vi "FRCts20_WebMethods_Convert_Request.vi"(8 "error in (no error)":errorcluster, 10 "Team Out":T8, 11 "Request Out":T9) -> (0 "error out":errorcluster, 3 "Request+Team":cluster{"Request":T1, "Team":T4})   [LabVIEW 2014, in "FRCts20_WebMethods.lvlib"]
uses:
  FRCts20_WebMethods.lvlib
  Backend/source/VI Source/FRCts20_Backend_API/FRCts20_Backend_API_Request.ctl
  Backend/source/VI Source/FRCts20_Backend_API/FRCts20_Backend_API_Status.ctl
  Backend/source/VI Source/FRCts20_Backend_API/FRCts20_Backend_API_Team.ctl
  Backend/source/VI Source/FRCts20_Backend_API/FRCts20_Backend_API_SW.ctl
  ESP Engine/source/VI Source/TypeDefs/FRCts20_EspEngine_Request.ctl
  Web Method Public Interface/FRCts20_WebMethods_ctl_request.ctl
  ESP Engine/source/VI Source/TypeDefs/FRCts20_EspEngine_Team.ctl
  Web Method Public Interface/FRCts20_WebMethods_ctl_singleTeam.ctl
  Web Method Public Interface/FRCts20_WebMethods_ctl_teamIdentifier.ctl
  ESP Engine/source/VI Source/FRCts20_EspEngine.lvlib
  Backend/source/VI Source/FRCts20_Backend_API/FRCts20_Backend_API.lvlib
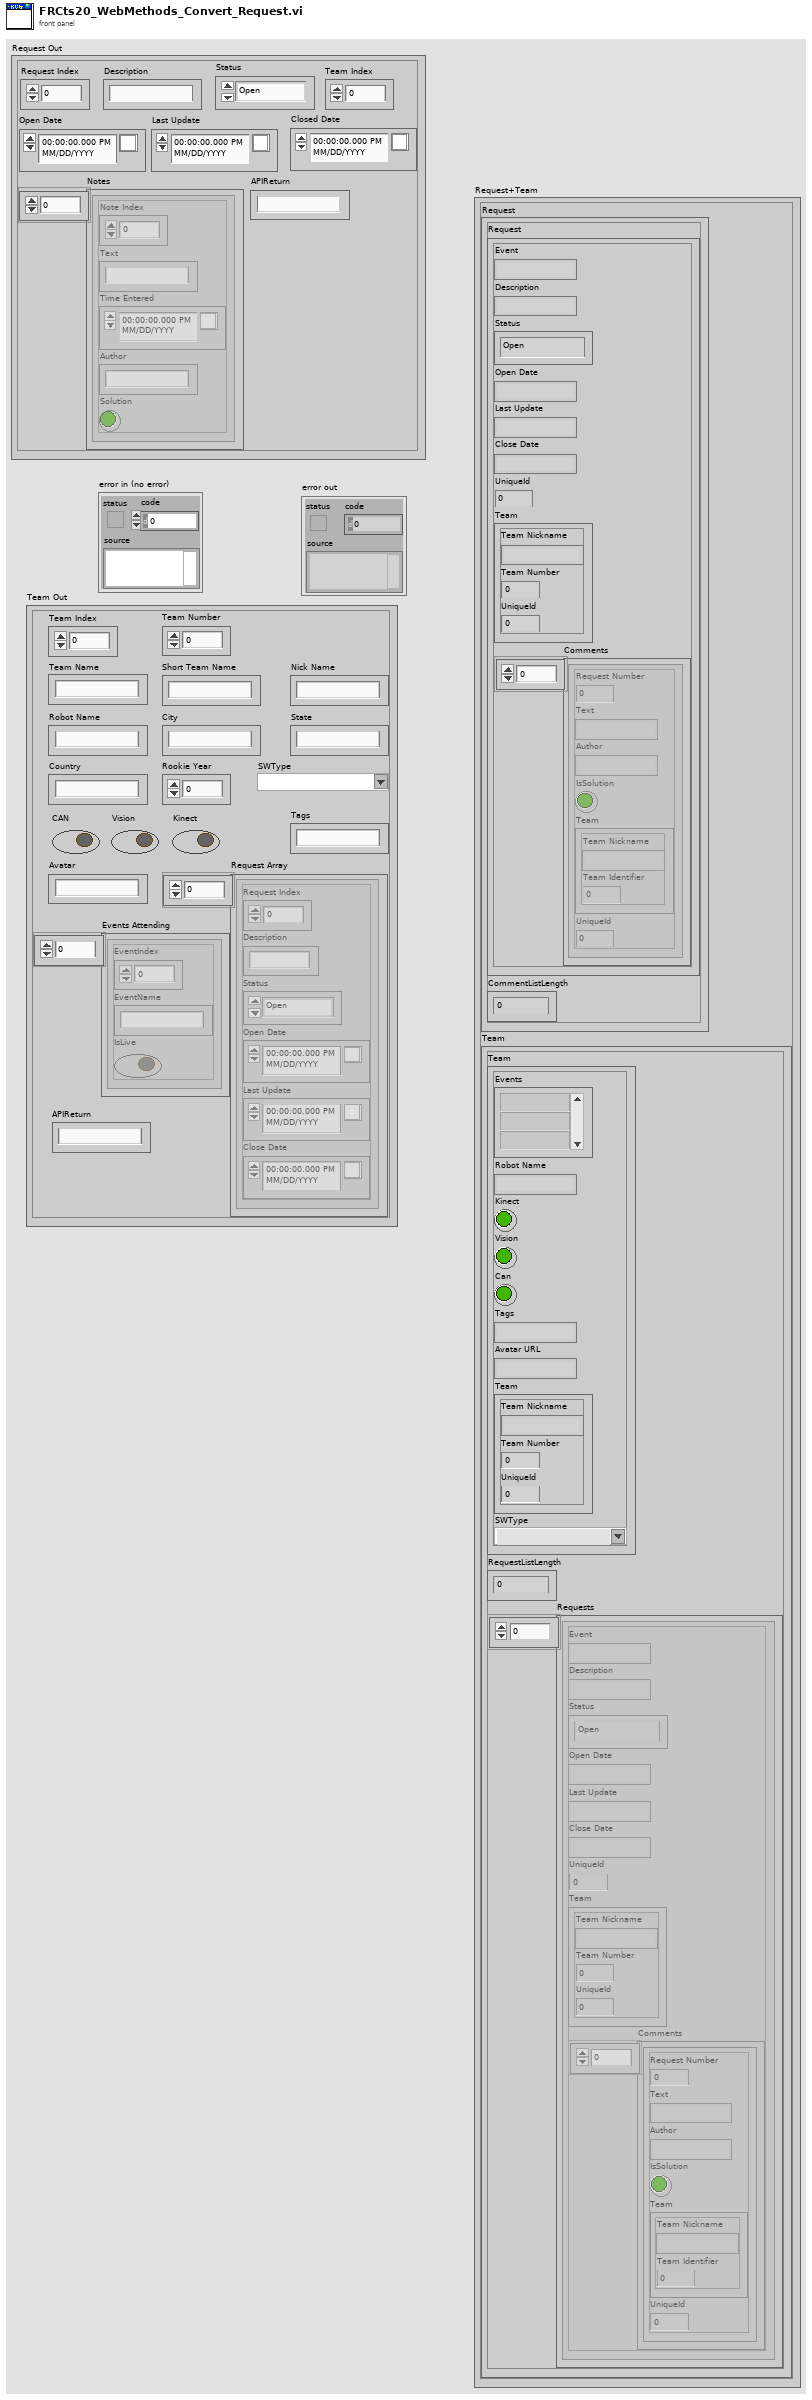
[diagram p1: front panel]
types:
  T1 = typedef "FRCts20_EspEngine.lvlib/FRCts20_EspEngine_Request.ctl" = cluster{"Request":T2, "CommentListLength":i16}
  T2 = typedef "FRCts20_WebMethods.lvlib/FRCts20_WebMethods_ctl_request.ctl" = cluster{"Event":string, "Description":string, "Status":T3, "Open Date":string, "Last Update":string, "Close Date":string, "UniqueId":i32, "Team":cluster{"Team Nickname":string, "Team Number ":i32, "UniqueId":i32}, "Comments":cluster{"Request Number":dbl, "Text":string, "Author":string, "IsSolution":bool, "Team":cluster{"Team Nickname":string, "Team Identifier ":dbl}, "UniqueId":i32}[]}
  T3 = typedef "FRCts20_Backend_Engine.lvlib/FRCts20_Backend_API.lvlib/FRCts20_Backend_API_Status.ctl" = enum16{"Open", "In Work", "Closed"}
  T4 = typedef "FRCts20_EspEngine.lvlib/FRCts20_EspEngine_Team.ctl" = cluster{"Team":T5, "RequestListLength":i16, "Requests":T2[]}
  T5 = typedef "FRCts20_WebMethods.lvlib/FRCts20_WebMethods_ctl_singleTeam.ctl" = cluster{"Events":string[], "Robot Name":string, "Kinect":bool, "Vision":bool, "Can":bool, "Tags":string, "Avatar URL":string, "Team":T6, "SWType":T7}
  T6 = typedef "FRCts20_WebMethods.lvlib/FRCts20_WebMethods_ctl_teamIdentifier.ctl" = cluster{"Team Nickname":string, "Team Number ":u32, "UniqueId":u32}
  T7 = typedef "FRCts20_Backend_Engine.lvlib/FRCts20_Backend_API.lvlib/FRCts20_Backend_API_SW.ctl" = string
  T8 = typedef "FRCts20_Backend_Engine.lvlib/FRCts20_Backend_API.lvlib/FRCts20_Backend_API_Team.ctl" = cluster{"Team Index":u32, "Team Number":u32, "Team Name":string, "Short Team Name":string, "Nick Name":string, "Robot Name":string, "City":string, "State":string, "Country":string, "Rookie Year":u32, "SWType":T7, "CAN":bool, "Vision":bool, "Kinect":bool, "Tags":string, "Avatar":string, "Request Array":cluster{"Request Index":u32, "Description":string, "Status":T3, "Open Date":timestamp, "Last Update":timestamp, "Close Date":timestamp}[], "Events Attending":cluster{"EventIndex":dbl, "EventName":string, "IsLive":bool}[], "APIReturn":string}
  T9 = typedef "FRCts20_Backend_Engine.lvlib/FRCts20_Backend_API.lvlib/FRCts20_Backend_API_Request.ctl" = cluster{"Request Index":u32, "Description":string, "Status":T3, "Open Date":timestamp, "Last Update":timestamp, "Closed Date":timestamp, "Notes":cluster{"Note Index":u32, "Text":string, "Time Entered":timestamp, "Author":string, "Solution":bool}[], "Team Index":u32, "APIReturn":string}
  T10 = cluster{"Request Number":dbl, "Text":string, "Author":string, "IsSolution":bool, "Team":cluster{"Team Nickname":string, "Team Identifier ":dbl}, "UniqueId":i32}
  T11 = cluster{"EventIndex":dbl, "EventName":string, "IsLive":bool}[]
  T12 = cluster{"Request Index":u32, "Description":string, "Status":T3, "Open Date":timestamp, "Last Update":timestamp, "Close Date":timestamp}[]
  T13 = cluster{"Note Index":u32, "Text":string, "Time Entered":timestamp, "Author":string, "Solution":bool}[]
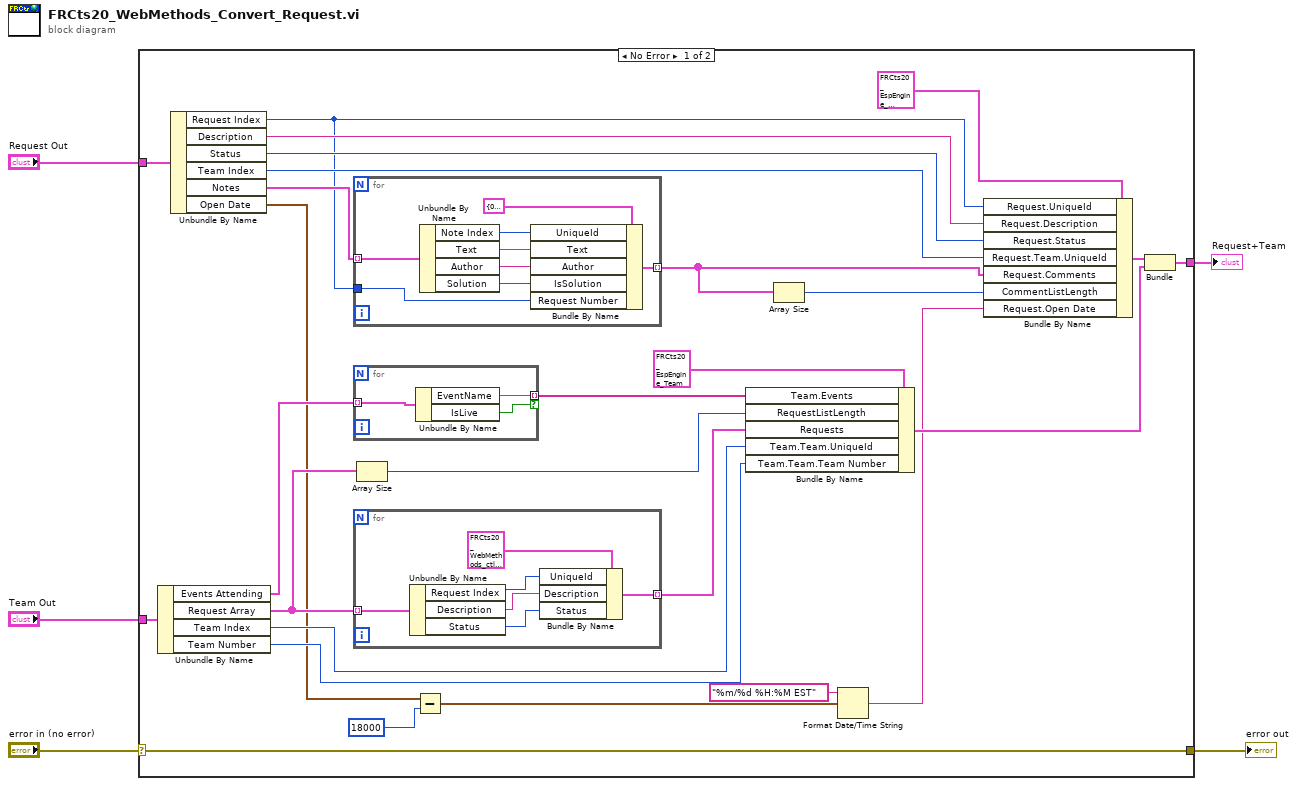
[diagram p0: block diagram]
diagram:
  n1 = case shown="No Error" "error in (no error)" {
    selector: "error in (no error)" -> [w23 w50]
    tunnel: [w23 w50] -> w5
    tunnel: "Request Out" -> [w24 _]
    tunnel: "Team Out" -> [w21 _]
    tunnel: [w15 _] -> w1
    frame No Error {
      n2 = Unbundle By Name(w21) -> ("Events Attending"=w12:T11, "Request Array"=w19:T12, "Team Index"=w14:u32, "Team Number"=w13:u32)
      n3 = Unbundle By Name(w24) -> ("Request Index"=w27:u32, "Description"=w31:string, "Status"=w30:T3, "Team Index"=w29:u32, "Notes"=w28:T13, "Open Date"=w9:timestamp)
      n4 = for {
        tunnel: [w48] -> w25 mode=indexing
        tunnel: w28 -> [w47] mode=indexing
        tunnel: w27 -> [w42]
        n5 = Unbundle By Name(w47) -> ("Note Index"=w46:u32, "Text"=w45:string, "Author"=w44:string, "Solution"=w43:bool)
        n6 = Bundle By Name(cluster=T10 {"Request Number"=0.0, "Text"="", "Author"="", "IsSolution"=FALSE, "Team"={"Team Nickname"="", "Team Identifier "=0.0}, "UniqueId"=0} ("Comment"), "UniqueId"=w46, "Text"=w45, "Author"=w44, "IsSolution"=w43, "Request Number"=w42) -> (w48:T10)
      }
      n7 = for {
        tunnel: w12 -> [w35] mode=indexing
        tunnel: [w34] -> w11 mode=indexing if=w33
        n8 = Unbundle By Name(w35) -> ("EventName"=w34:string, "IsLive"=w33:bool)
      }
      n9 = for {
        tunnel: w19 -> [w41] mode=indexing
        tunnel: [w37] -> w18 mode=indexing
        n10 = Unbundle By Name(w41) -> ("Request Index"=w39:u32, "Description"=w38:string, "Status"=w36:T3)
        n11 = Bundle By Name(cluster=T2 {"Event"="", "Description"="", "Status"=enum."Open", "Open Date"="", "Last Update"="", "Close Date"="", "UniqueId"=0, "Team"={"Team Nickname"="", "Team Number "=0, "UniqueId"=0}, "Comments"=[]} ("Request"), "UniqueId"=w39, "Description"=w38, "Status"=w36) -> (w37:T2)
      }
      n12 = Array Size(array=w19) -> (size(s)=w20:i32)
      n13 = Subtract(x=w9, y=18000) -> (x-y=w8:timestamp)
      n14 = Bundle By Name(cluster=T4 {"Team"={"Events"=[], "Robot Name"="", "Kinect"=FALSE, "Vision"=FALSE, "Can"=FALSE, "Tags"="", "Avatar URL"="", "Team"={"Team Nickname"="", "Team Number "=0, "UniqueId"=0}, "SWType"=""}, "RequestListLength"=0, "Requests"=[]} ("Team"), "Team.Events"=w11, "RequestListLength"=w20, "Requests"=w18, "Team.Team.UniqueId"=w14, "Team.Team.Team Number"=w13) -> (w16:T4)
      n15 = Array Size(array=w25) -> (size(s)=w26:i32)
      n16 = Format Date/Time String(time format string (%c)="%m/%d %H:%M EST", seconds (now)=w8) -> (date/time string=w10:string)  [unwired: 1 in]
      n17 = Bundle By Name(cluster=T1 {"Request"={"Event"="", "Description"="", "Status"=enum."Open", "Open Date"="", "Last Update"="", "Close Date"="", "UniqueId"=0, "Team"={"Team Nickname"="", "Team Number "=0, "UniqueId"=0}, "Comments"=[]}, "CommentListLength"=0} ("Request"), "Request.UniqueId"=w27, "Request.Description"=w31, "Request.Status"=w30, "Request.Team.UniqueId"=w29, "Request.Comments"=w25, "CommentListLength"=w26, "Request.Open Date"=w10) -> (w17:T1)
      n18 = Bundle("Request"=w17, "Team"=w16) -> (w15:cluster{"Request":T1, "Team":T4})  [unwired: 1 in]
    }
    frame Error {
    }
  }
  "error out" <- w5
  "Request+Team" <- w1
